vi "ToXYGraph.vi"(8 "error in":errorcluster, 11 "Generic in":refnum<class "Generic.lvclass">) -> (0 "error out":errorcluster, 3 "XYGraph out":refnum<class "XYGraph.lvclass">)   [LabVIEW 2014, in "XYGraph.lvclass"]
uses:
  XYGraph.lvclass
  Generic/Generic.lvclass
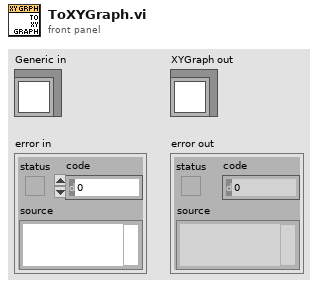
[diagram p1: front panel]
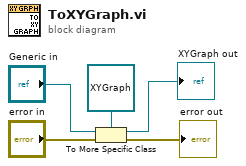
[diagram p0: block diagram]
diagram:
  n1 = To More Specific Class(target class=refnum<class "XYGraph.lvclass"> refnum ("RotaryColorScale in 2"), reference="Generic in", error in="error in") -> (specific class reference=→"XYGraph out":refnum<class "XYGraph.lvclass">, error out=→"error out":errorcluster)
